vi "SetTriggerMode.vi"(8 "Error In":errorcluster, 9 "Trigger Mode":T1, 10 "Line (1-14)":u8=1 min=1 max=14 step=1, 11 "Keithley 2602 In":refnum<visa-resource-name>) -> (0 "Error Out":errorcluster, 3 "Keithley 2602 Out":refnum<visa-resource-name>)   [LabVIEW 2012, in "Keithley-2602.lvlib"]
uses:
  Keithley-2602.lvlib
  Controls/TriggerMode.ctl
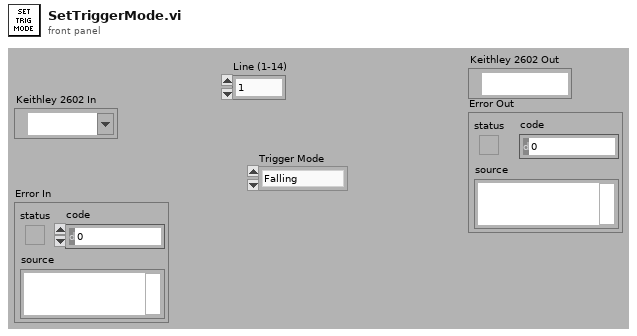
[diagram p1: front panel]
types:
  T1 = typedef "Keithley-2602.lvlib/TriggerMode.ctl" = enum16{"Falling", "Rising", "Either", "Synchronous"}
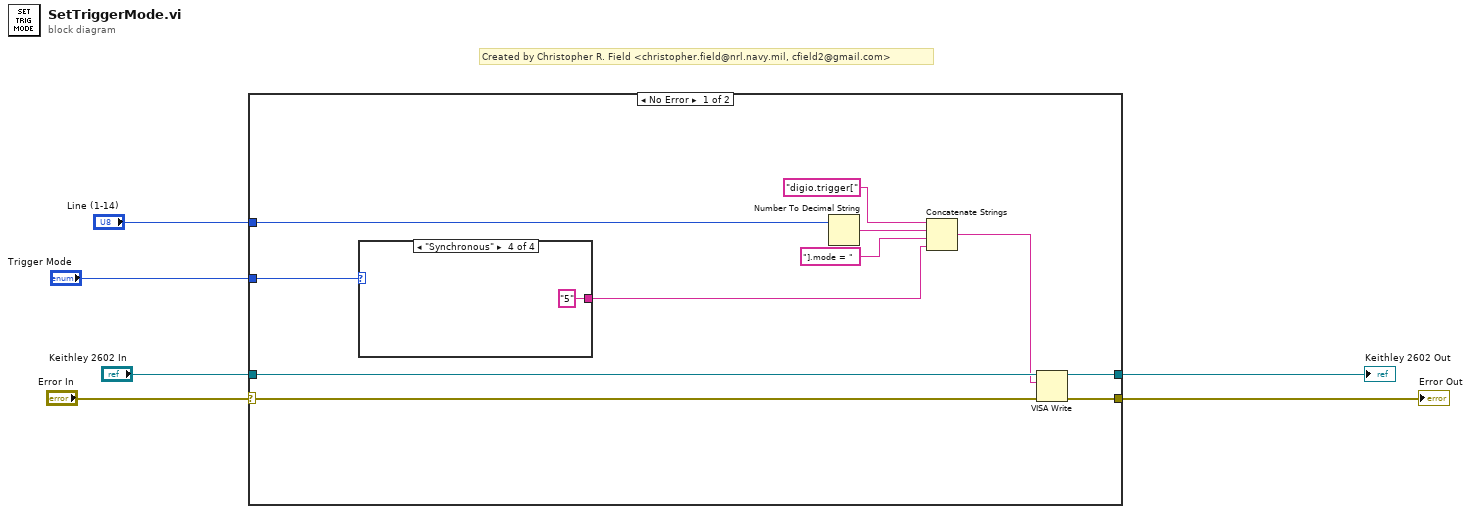
[diagram p0: block diagram]
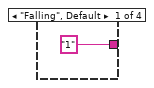
[diagram p2: hidden frame]
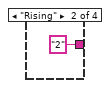
[diagram p3: hidden frame]
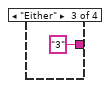
[diagram p4: hidden frame]
diagram:
  # "Created by Christopher R. Field <christopher.field@nrl.navy.mil, cfield2@gmail.com>"
  n1 = case shown="No Error" "Error In" {
    selector: "Error In" -> [w9 w22]
    tunnel: "Keithley 2602 In" -> [w17 w23]
    tunnel: [w16 w23] -> w5
    tunnel: [w15 w22] -> w4
    tunnel: "Line (1-14)" -> [w14 _]
    tunnel: "Trigger Mode" -> [w8 _]
    frame No Error {
      n2 = case shown="\"Synchronous\"" w8 {
        tunnel: ["1" "2" "3" "5"] -> w7
        frame "Falling", Default {
        }
        frame "Rising" {
        }
        frame "Either" {
        }
        frame "Synchronous" {
        }
      }
      n3 = Number To Decimal String(number=w14) -> (decimal integer string=w12:string)  [unwired: 1 in]
      n4 = Concatenate Strings("digio.trigger[", w12, "].mode = ", w7) -> (w10:string)
      n5 = VISA Write(VISA resource name=w17, write buffer=w10, error in (no error)=w9) -> (VISA resource name out=w16:refnum<visa-resource-name>, error out=w15:errorcluster)  [unwired: 1 out]
    }
    frame Error {
    }
  }
  "Keithley 2602 Out" <- w5
  "Error Out" <- w4
